vi "Create_Pos_array.vi"(2 "Traverse line":T1 {"Row Duration (mins)" format="%#.1f"; "Row No" min=0; "Trace Gas Concentration (%)" min=0.0 format="%#.2f"; "Emission Rate (l/min)" format="%#.2f"; "Tunnel Speed" format="%#.2f"; "Start X" format="%#.2f"; "Start Y" format="%#.2f"; "Start Z" format="%#.2f"; "End X" format="%#.2f"; "End Y" format="%#.2f"; "End Z" format="%#.2f"; "Averaging time (min)" min=0.0 format="%#.2f"}) -> (5 "Traverse line Out":T1 {"Row Duration (mins)" format="%#.1f"; "Row No" min=0; "Trace Gas Concentration (%)" min=0.0 format="%#.2f"; "Emission Rate (l/min)" format="%#.2f"; "Tunnel Speed" format="%#.2f"; "Start X" format="%#.2f"; "Start Y" format="%#.2f"; "Start Z" format="%#.2f"; "End X" format="%#.2f"; "End Y" format="%#.2f"; "End Z" format="%#.2f"; "Averaging time (min)" min=0.0 format="%#.2f"}, 6 "Error Messages":string, 7 "Array of Positions":dbl[][](array[numeric]) format="%.2f", 9 "Axis Traversed":enum16{"X traverse", "Y traverse", "Z traverse"}(ring))   [LabVIEW 2010]
uses:
  Traverse_cluster.ctl
  Spacing.ctl
  Controls/Multi_run_mode.ctl
  Globals/Extra_Commands_Global.vi
panel:
  # "X           Y            Z"
  # "Start"
  # "End"
  # "X           Y            Z"
  # "Start"
  # "End"
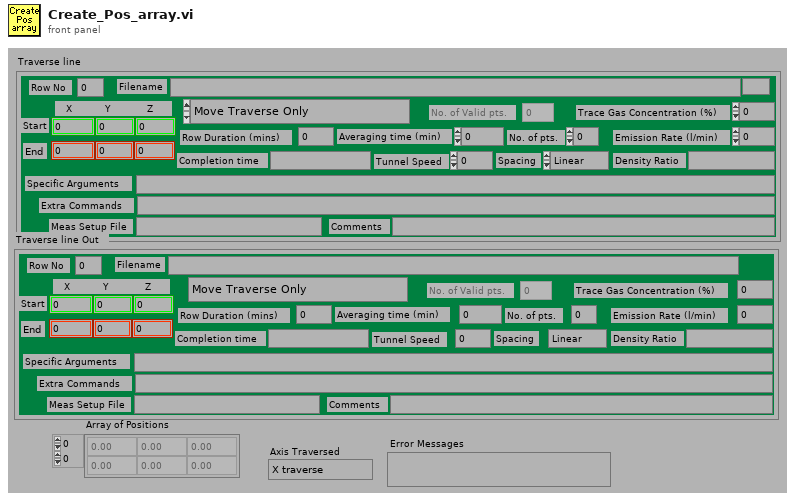
[diagram p1: front panel]
types:
  T1 = typedef "Traverse_cluster.ctl" = cluster{"Start X":dbl, "Start Y":dbl, "Start Z":dbl, "End X":dbl, "End Y":dbl, "End Z":dbl, "No. of pts.":i32, "Spacing":T2, "Filename":path, "Tunnel Speed":dbl, "Averaging time (min)":dbl, "Extra Commands":string, "Specific Arguments":string, "Emission Rate (l/min)":dbl, "Trace Gas Concentration (%)":dbl, "Density Ratio":string, "Comments":string, "Row No":i32, "Row Type Selector":T3, "Completion time":string, "Row Duration (mins)":dbl, "No. of Valid pts.":i32, "Meas Setup File":string}
  T2 = typedef "Spacing.ctl" = enum16{"Linear", "Log", "Gauss", "Specified", "N/A"}
  T3 = typedef "Multi_run_mode.ctl" = enum16{"Move Traverse Only", "Set Tunnel Speed Only", "Set Source Only", "Set Measurement Conditions", "Single Measurement", "Vertical Profile", "Lateral Profile", "Longitudinal Profile", "Explore Volume", "Multi-Axis Profile", "Auto Calibrate", "Meas Fast FID Bkgnd", "Check Beam Power", "Scanning Valve Measurement", "Run VI Named:", "Set ADAM Ch", "Wait (minutes)", "Send Message", "Synchronize With:", "Fall Back to this Row", "Turn Off Row Repeating", "Blank Row"}
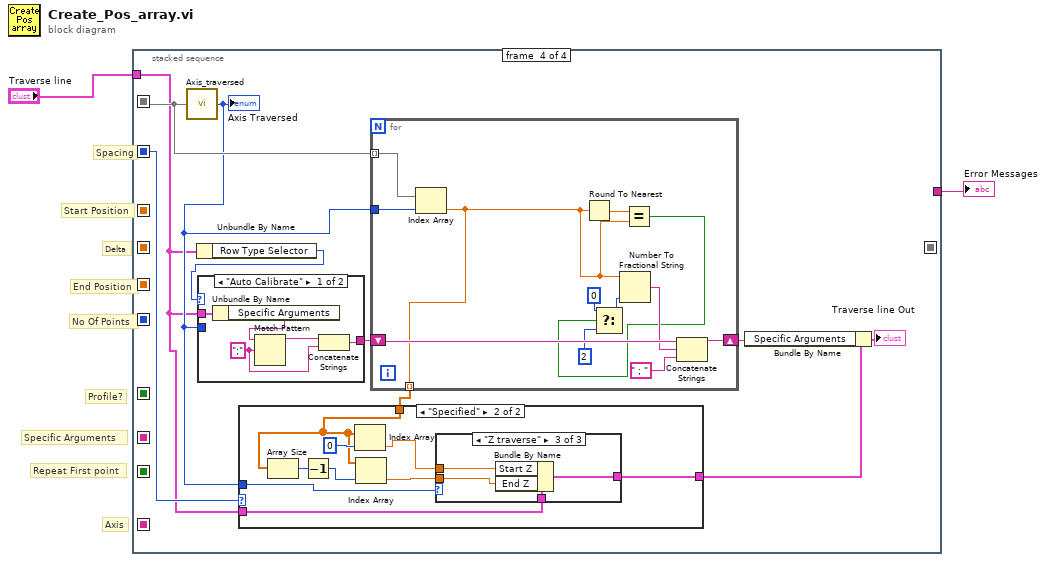
[diagram p0: block diagram]
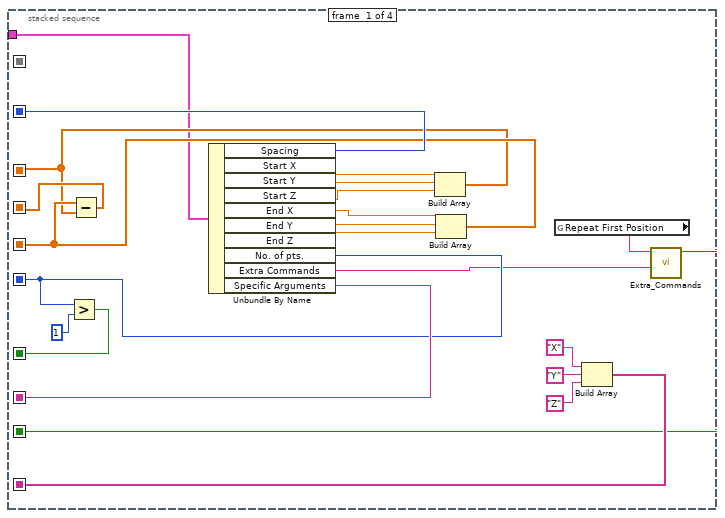
[diagram p2: hidden frame]
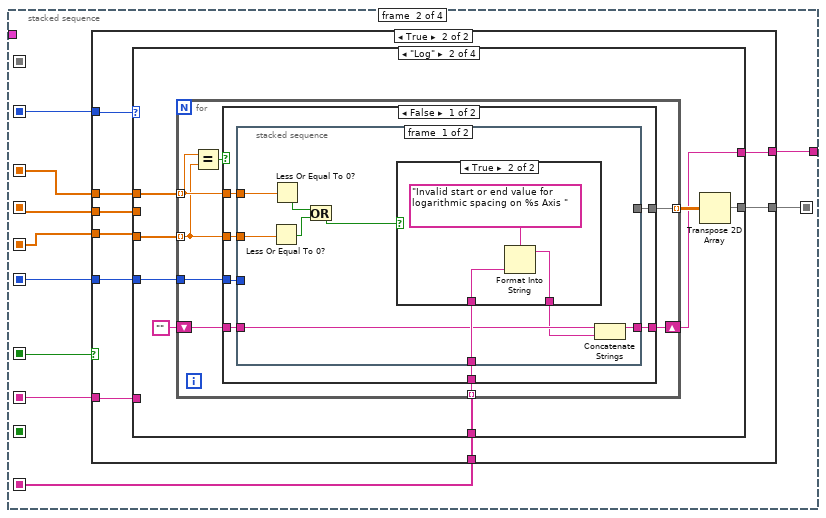
[diagram p3: hidden frame]
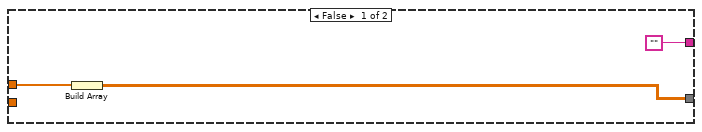
[diagram p4: hidden frame]
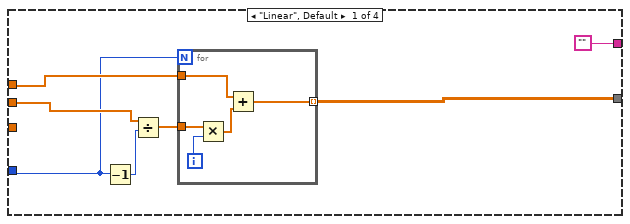
[diagram p5: hidden frame]
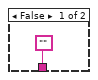
[diagram p6: hidden frame]
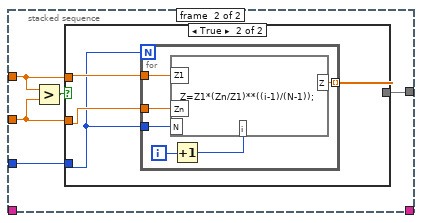
[diagram p7: hidden frame]
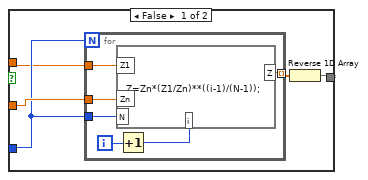
[diagram p8: hidden frame]
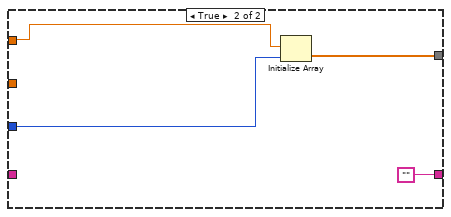
[diagram p9: hidden frame]
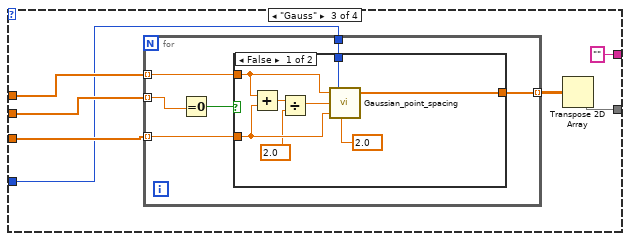
[diagram p10: hidden frame]
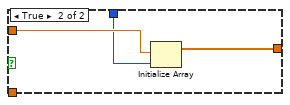
[diagram p11: hidden frame]
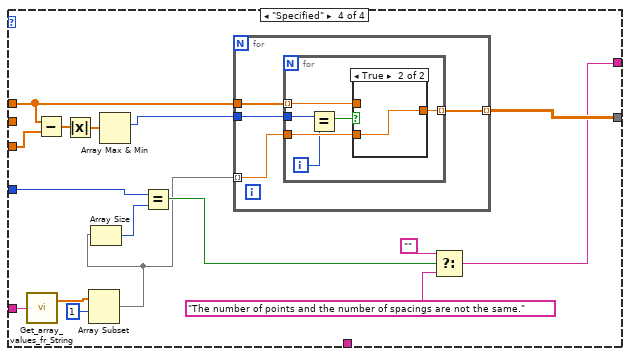
[diagram p12: hidden frame]
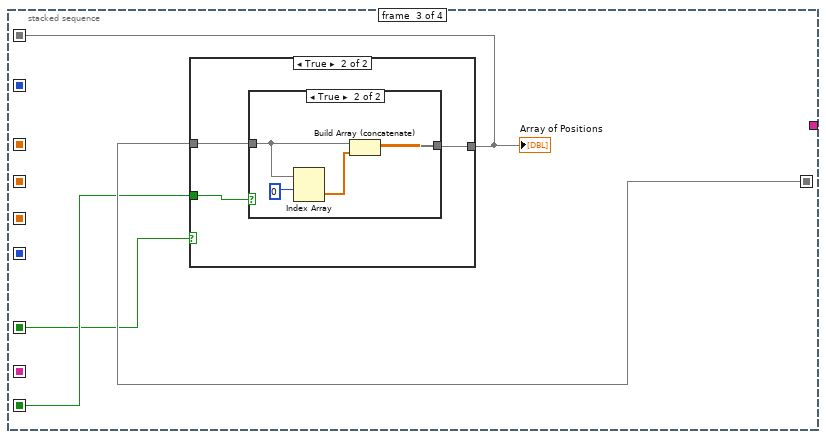
[diagram p14: hidden frame]
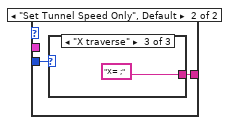
[diagram p17: hidden frame]
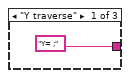
[diagram p18: hidden frame]
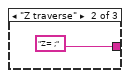
[diagram p19: hidden frame]
diagram:
  # "Axis"
  # "Profile?"
  # "Delta"
  # "Repeat First point"
  # "Spacing"
  # "No Of Points"
  # "Specific Arguments"
  # "End Position"
  # "Start Position"
  n1 = stacked-sequence {
    seq-local: [_ w34 _ _] -> [_ _ w180 _]
    seq-local: [w11 _ _ _] -> [_ w31 _ _]
    seq-local: [w16 _ _ _] -> [_ w29 _ _]
    seq-local: [w17 _ _ _] -> [_ w30 _ _]
    seq-local: [w13 _ _ _] -> [_ w27 _ _]
    seq-local: [w15 _ _ _] -> [_ w33 _ _]
    seq-local: [w24 _ _ _] -> [_ w32 _ w195]
    seq-local: [w4 _ _ _] -> [_ _ w179 _]
    seq-local: [w12 _ _ _] -> [_ w26 w178 _]
    seq-local: [w7 _ _ _] -> [_ w25 _ _]
    seq-local: [_ _ w177 _] -> [_ _ _ w199]
    tunnel: [_ w28 _ _] -> w2
    tunnel: "Traverse line" -> [w3 _ _ w190]
    frame #0 {
      n2 = Unbundle By Name(w3) -> ("Spacing"=w24:T2, "Start X"=w23:dbl, "Start Y"=w22:dbl, "Start Z"=w21:dbl, "End X"=w20:dbl, "End Y"=w19:dbl, "End Z"=w18:dbl, "No. of pts."=w13:i32, "Extra Commands"=w5:string, "Specific Arguments"=w15:string)
      n3 = Greater?(x=w13, y=1) -> (0:w12:bool)
      n4 = Build Array(w23, w22, w21) -> (w11:dbl[])
      n5 = Build Array(w20, w19, w18) -> (w17:dbl[])
      n6 = Subtract(x=w17, y=w11) -> (x-y=w16:dbl[])
      n7 = global read "Extra_Commands_Global.vi" "Repeat First Position"() -> (w6:string)
      n8 = Build Array("X", "Y", "Z") -> (w7:string[])
      n9 = call "Extra_Commands.vi"("String to Search"=w5, "Command"=w6) -> ("Command Found"=w4:bool)  [unwired: 1 in, 4 out]
    }
    frame #1 {
      n10 = case shown="True" w26 {
        tunnel: [w36 w46] -> w34
        tunnel: w33 -> [_ w45]
        tunnel: w32 -> [_ w44]
        tunnel: w31 -> [w37 w43]
        tunnel: w30 -> [_ w42]
        tunnel: w29 -> [_ w41]
        tunnel: w27 -> [_ w40]
        tunnel: ["" w39] -> w28
        tunnel: w25 -> [_ w38]
        frame False {
          n11 = Build Array(w37) -> (w36:dbl[][])
        }
        frame True {
          n12 = case shown="\"Log\"" w44 {
            tunnel: w42 -> [_ w64 w129 w156]
            tunnel: w43 -> [w52 w65 w130 w152]
            tunnel: w40 -> [w50 w66 w128 w161]
            tunnel: [w53 w63 w127 w163] -> w46
            tunnel: w41 -> [w51 _ w131 _]
            tunnel: w45 -> [_ _ _ w164]
            tunnel: ["" w59 "" ("f") w157] -> w39
            tunnel: w38 -> [_ w61 _ _]
            frame "Linear", Default {
              n13 = Decrement(x=w50) -> (x-1=w48:i32)
              n14 = Divide(x=w51, y=w48) -> (x/y=w49:dbl[])
              n15 = for {
                N: w50 -> [_]
                tunnel: w49 -> [w57]
                tunnel: w52 -> [w55]
                tunnel: [w54] -> w53 mode=indexing
                i -> [w58]
                n16 = Multiply(x=w57, y=w58) -> (x*y=w56:dbl[])
                n17 = Add(x=w55, y=w56) -> (x+y=w54:dbl[])
              }
            }
            frame "Log" {
              n18 = for {
                tunnel: [w74] -> w62 mode=indexing
                tunnel: w65 -> [w72] mode=indexing
                tunnel: w64 -> [w71] mode=indexing
                tunnel: w66 -> [w73]
                tunnel: w61 -> [w69] mode=indexing
                shift-right: [w67] -> w59
                shift-left: "" -> [w68]
                n19 = Equal?(x=w72, y=w71) -> (x = y?=w70:bool)
                n20 = case shown="False" w70 {
                  tunnel: w73 -> [w81 w123]
                  tunnel: w71 -> [w80 _]
                  tunnel: w72 -> [w79 w122]
                  tunnel: [w78 w124] -> w74
                  tunnel: w69 -> [w77 _]
                  tunnel: w68 -> [w76 _]
                  tunnel: [w75 ""] -> w67
                  frame False {
                    n21 = stacked-sequence {
                      tunnel: [_ w98] -> w78
                      tunnel: w79 -> [w90 w97]
                      tunnel: w80 -> [w89 w96]
                      tunnel: w81 -> [_ w95]
                      tunnel: w77 -> [w85 _]
                      tunnel: w76 -> [w84 _]
                      tunnel: [w82 _] -> w75
                      frame #0 {
                        n22 = Less Or Equal To 0?(x=w89) -> (x <= 0?=w88:bool)
                        n23 = Less Or Equal To 0?(x=w90) -> (x <= 0?=w87:bool)
                        n24 = Or(x=w87, y=w88) -> (x .or. y?=w86:bool)
                        n25 = case shown="True" w86 {
                          tunnel: w85 -> [_ w94]
                          tunnel: ["" w92] -> w83
                          frame False {
                          }
                          frame True {
                            n26 = Format Into String(format string="Invalid start or end value for logarithmic spacing on %s Axis " ("Format String"), w94) -> (resulting string=w92:string)  [unwired: 2 in, 1 out]
                          }
                        }
                        n27 = Concatenate Strings(w84, w83) -> (w82:string)
                      }
                      frame #1 {
                        n28 = Greater?(x=w97, y=w96) -> (0:w99:bool)
                        n29 = case shown="True" w99 {
                          tunnel: [w101 w111] -> w98
                          tunnel: w97 -> [w100 w114]
                          tunnel: w96 -> [w104 w113]
                          tunnel: w95 -> [w103 w112]
                          frame False {
                            n30 = for {
                              N: w103 -> [_]
                              tunnel: w104 -> [w107]
                              tunnel: w103 -> [w106]
                              tunnel: [w108] -> w102 mode=indexing
                              tunnel: w100 -> [w105]
                              i -> [w110]
                              n31 = Increment(x=w110) -> (x+1=w109:i32)
                              n32 = formula code="Z=Zn*(Z1/Zn)**((i-1)/(N-1));"("i"=w109, "N"=w106, "Zn"=w107, "Z1"=w105) -> ("Z"=w108:dbl)
                            }
                            n33 = Reverse 1D Array(array=w102) -> (reversed array=w101:dbl[])
                          }
                          frame True {
                            n34 = for {
                              N: w112 -> [_]
                              tunnel: w114 -> [w120]
                              tunnel: w113 -> [w119]
                              tunnel: w112 -> [w116]
                              tunnel: [w115] -> w111 mode=indexing
                              i -> [w118]
                              n35 = Increment(x=w118) -> (x+1=w117:i32)
                              n36 = formula code="Z=Z1*(Zn/Z1)**((i-1)/(N-1));"("i"=w117, "N"=w116, "Zn"=w119, "Z1"=w120) -> ("Z"=w115:dbl)
                            }
                          }
                        }
                      }
                    }
                  }
                  frame True {
                    n37 = Initialize Array(w122, w123) -> (w124:dbl[])
                  }
                }
              }
              n38 = Transpose 2D Array(2D array=w62) -> (transposed array=w63:dbl[][])
            }
            frame "Gauss" {
              n39 = for {
                tunnel: w131 -> [w137] mode=indexing
                tunnel: w130 -> [w135] mode=indexing
                tunnel: w129 -> [w134] mode=indexing
                tunnel: w128 -> [w133]
                tunnel: [w132] -> w126 mode=indexing
                n40 = Equal To 0?(x=w137) -> (x = 0?=w136:bool)
                n41 = case shown="False" w136 {
                  tunnel: w135 -> [w142 w148]
                  tunnel: w134 -> [w141 _]
                  tunnel: w133 -> [w145 w147]
                  tunnel: [w144 w146] -> w132
                  frame False {
                    n42 = Add(x=w142, y=w141) -> (x+y=w140:dbl)
                    n43 = Divide(x=w140, y=2.0) -> (x/y=w138:dbl)
                    n44 = call "Gaussian_point_spacing.vi"("Start point"=w142, "No of points"=w145, "Centre point"=w138, "End point"=w141, "Guass intensity"=2.0) -> ("Positions"=w144:dbl[])  [unwired: 2 out]
                  }
                  frame True {
                    n45 = Initialize Array(w148, w147) -> (w146:dbl[])
                  }
                }
              }
              n46 = Transpose 2D Array(2D array=w126) -> (transposed array=w127:dbl[][])
            }
            frame "Specified" {
              n47 = call "Get_array_values_fr_String.vi"("String Value"=w164) -> ("Numeric Array"=w151:dbl[])  [unwired: 1 out]
              n48 = Subtract(x=w152, y=w156) -> (x-y=w155:dbl[])
              n49 = Absolute Value(x=w155) -> (abs(x)=w154:dbl[])
              n50 = Array Subset(array=w151, index=1) -> (w149:dbl[])  [unwired: 1 in]
              n51 = Array Size(array=w149) -> (size(s)=w162:i32)
              n52 = Array Max & Min(array=w154) -> (max index (indices)=w153:i32)  [unwired: 3 out]
              n53 = Equal?(x=w161, y=w162) -> (x = y?=w160:bool)
              n54 = for {
                tunnel: w149 -> [w166] mode=indexing
                tunnel: [w167] -> w163 mode=indexing
                tunnel: w153 -> [w168]
                tunnel: w152 -> [w165]
                n55 = for {
                  tunnel: w168 -> [w172]
                  tunnel: [w174] -> w167 mode=indexing
                  tunnel: w166 -> [w173]
                  tunnel: w165 -> [w169] mode=indexing
                  i -> [w171]
                  n56 = Equal?(x=w172, y=w171) -> (x = y?=w170:bool)
                  n57 = case shown="True" w170 {
                    tunnel: [w175 w176] -> w174
                    tunnel: w173 -> [_ w176]
                    tunnel: w169 -> [w175 _]
                    frame False {
                    }
                    frame True {
                    }
                  }
                }
              }
              n58 = Select(t="", s=w160, f="The number of points and the number of spacings are not the same.") -> (s? t:f=w157:string)
            }
          }
        }
      }
    }
    frame #2 {
      n59 = case shown="True" w178 {
        tunnel: [w181 w184] -> w177
        tunnel: w180 -> [w181 w183]
        tunnel: w179 -> [_ w182]
        frame False {
        }
        frame True {
          n60 = case shown="True" w182 {
            tunnel: [w185 w189] -> w184
            tunnel: w183 -> [w185 w187]
            frame False {
            }
            frame True {
              n61 = Index Array(array=w187, index (row)=0) -> (element=w188:dbl[])  [unwired: 1 in]
              n62 = Build Array (concatenate)(w187, w188) -> (w189:dbl[][])
            }
          }
        }
      }
      "Array of Positions" <- w177
    }
    frame #3 {
      n63 = call "Axis_traversed.vi"("Position array"=w199) -> ("Axis Traversed"=w193:enum16{"X traverse", "Y traverse", "Z traverse"})  [unwired: 4 out]
      "Axis Traversed" <- w193
      n64 = Unbundle By Name(w190) -> ("Row Type Selector"=w191:T3)
      n65 = case shown="\"Auto Calibrate\"" w191 {
        tunnel: [w202 w206] -> w196
        tunnel: w193 -> [_ w205]
        tunnel: w190 -> [w204 _]
        frame "Auto Calibrate" {
          w200 = ";" ("regular expression")
          n66 = Unbundle By Name(w204) -> ("Specific Arguments"=w203:string)
          n67 = Match Pattern(string=w203, regular expression=w200) -> (before substring=w201:string)  [unwired: 4 out]
          n68 = Concatenate Strings(w201, w200) -> (w202:string)
        }
        frame "Set Tunnel Speed Only", Default {
          n69 = case shown="\"X traverse\"" w205 {
            tunnel: ["Y= ;" "Z= ;" "X= ;"] -> w206
            frame "Y traverse" {
            }
            frame "Z traverse" {
            }
            frame "X traverse" {
            }
          }
        }
      }
      n70 = for {
        tunnel: w193 -> [w243]
        tunnel: w199 -> [w233] mode=indexing
        shift-right: [w241] -> w198
        shift-left: w196 -> [w242]
        tunnel: [w232] -> w194 mode=indexing
        n71 = Index Array(array=w233, index=w243) -> (element=w232:dbl)
        n72 = Round To Nearest(number=w232) -> (nearest integer value=w235:dbl)
        n73 = Equal?(x=w235, y=w232) -> (x = y?=w234:bool)
        n74 = Select(t=0, s=w234, f=2) -> (s? t:f=w238:i32)
        n75 = Number To Fractional String(number=w232, precision (6)=w238) -> (F-format string=w240:string)  [unwired: 2 out]
        n76 = Concatenate Strings(w242, w240, " ; " ("string")) -> (w241:string)
      }
      n77 = case shown="\"Specified\"" w195 {
        tunnel: w194 -> [_ w214]
        tunnel: w193 -> [_ w219]
        tunnel: w190 -> [w210 w218]
        tunnel: [w210 w213] -> w192
        frame "Linear", Default {
        }
        frame "Specified" {
          n78 = Array Size(array=w214) -> (size(s)=w217:i32)
          n79 = Decrement(x=w217) -> (x-1=w215:i32)
          n80 = Index Array(array=w214, index=0) -> (element=w212:dbl)
          n81 = Index Array(array=w214, index=w215) -> (element=w211:dbl)
          n82 = case shown="\"Z traverse\"" w219 {
            tunnel: w218 -> [w223 w227 w231]
            tunnel: [w222 w226 w230] -> w213
            tunnel: w212 -> [w221 w225 w229]
            tunnel: w211 -> [w220 w224 w228]
            frame "X traverse" {
              n83 = Bundle By Name(cluster=w223, "Start X"=w221, "End X"=w220) -> (w222:T1)
            }
            frame "Y traverse" {
              n84 = Bundle By Name(cluster=w227, "Start Y"=w225, "End Y"=w224) -> (w226:T1)
            }
            frame "Z traverse" {
              n85 = Bundle By Name(cluster=w231, "Start Z"=w229, "End Z"=w228) -> (w230:T1)
            }
          }
        }
      }
      n86 = Bundle By Name(cluster=w192, "Specific Arguments"=w198) -> (→"Traverse line Out":T1)
    }
  }
  "Error Messages" <- w2
